vi "Close.vi"(8 "error in (no error)":errorcluster caption="entrée d'erreur (pas d'erreur)", 11 "Class DIO (Default) en entrée":refnum<class "Class Ana NI.lvclass">) -> (0 "error out":errorcluster caption="sortie d'erreur", 3 "Class DIO (Default) en sortie":refnum<class "Class Ana NI.lvclass">)   [LabVIEW 2020, in "Library Instrument & Equipement.lvlib" / "Library Ana.lvlib" / "Class Ana NI.lvclass"]
uses:
  Class Ana NI.lvclass
  Class Ana NI.lvclass/Class Ana NI.ctl
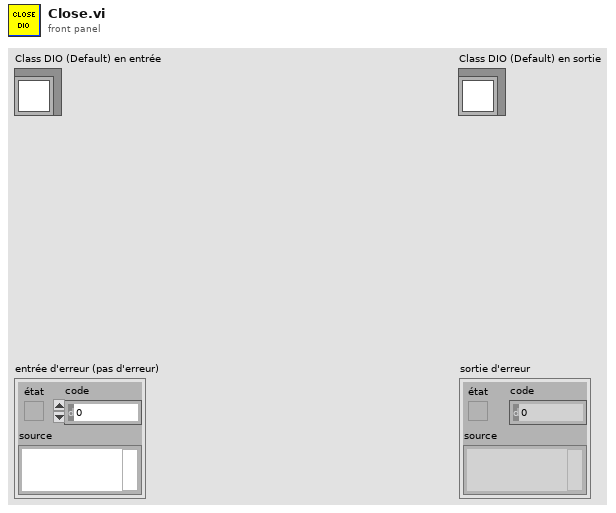
[diagram p1: front panel]
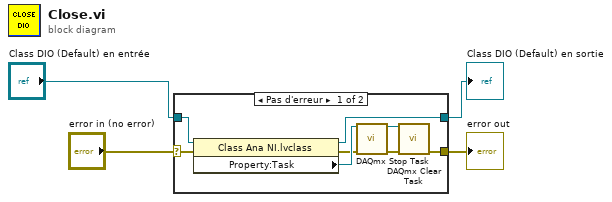
[diagram p0: block diagram]
diagram:
  n1 = case shown="Pas d'erreur" "error in (no error)" {
    selector: "error in (no error)" -> [w10 w14]
    tunnel: [w9 w14] -> w3
    tunnel: [w11 w13] -> w1
    tunnel: "Class DIO (Default) en entrée" -> [w12 w13]
    frame No Error {
      n2 = property class="Class Ana NI.lvclass"(reference=w12, error in=w10) -> (reference out=w11:refnum<class "Class Ana NI.lvclass">, error out=w6:errorcluster, "Property:Task"=w8:refnum<k21>)
      n3 = call <vilib>:"DAQmx Stop Task.vi"("task/channels in"=w8, "error in"=w6) -> ("task out"=w7:refnum<k21>, "error out"=w5:errorcluster)  [unwired: 12 in]
      n4 = call <vilib>:"DAQmx Clear Task.vi"("task in"=w7, "error in"=w5) -> ("error out"=w9:errorcluster)  [unwired: 13 in]
    }
    frame Error {
    }
  }
  "error out" <- w3
  "Class DIO (Default) en sortie" <- w1
